vi "Drum SubviUpdated.vi"(8 "Image Dst Out":T2, 14 "error out":errorcluster) -> (7 "Red Drum":bool, 9 "Yellow Array":bool[](array[boolean]), 13 "Foot Pedal":bool, 16 "Blue array":bool[](array[boolean]), 17 "Red Array":bool[](array[boolean]), 20 "Green Array":bool[](array[boolean]), 23 "Blue Drum 2":bool, 24 "Yellow Drum":bool, 25 "Green Drum":bool, 27 "error out 2":errorcluster)   [LabVIEW 2009]
uses:
  <vilib>/vision/Image Controls.llb/IMAQ Image.ctl
  <vilib>/Analysis/3filter.llb/Filter Passband Type.ctl
  <vilib>/Analysis/3filter.llb/Butterworth Filter (DBL).vi
  <vilib>/Analysis/NI_AALBase.lvlib
  <vilib>/vision/NI_Vision_Development_Module.lvlib
panel:
  in  "Yellow Drum":T1={"Global Rectangle"=[40, 272, 657, 396], "Contours"=[{"ID"=enum."External", "Type"=3, "Coordinates"=[40, 272, 657, 396]}]} {"Contours"."Type" items=["No Selection", "Point", "Line", "Rectangle", "Oval", "Polygon", "Freehand Region", "Annulus", "Unused2", "Unused3", "Broken Line", "Freehand Line", "Rotated Rectangle"]}
  in  "Red Drum":T1={"Global Rectangle"=[40, 272, 657, 396], "Contours"=[{"ID"=enum."External", "Type"=3, "Coordinates"=[40, 272, 657, 396]}]} {"Contours"."Type" items=["No Selection", "Point", "Line", "Rectangle", "Oval", "Polygon", "Freehand Region", "Annulus", "Unused2", "Unused3", "Broken Line", "Freehand Line", "Rotated Rectangle"]}
  in  "Green Drum":T1={"Global Rectangle"=[40, 272, 657, 396], "Contours"=[{"ID"=enum."External", "Type"=3, "Coordinates"=[40, 272, 657, 396]}]} {"Contours"."Type" items=["No Selection", "Point", "Line", "Rectangle", "Oval", "Polygon", "Freehand Region", "Annulus", "Unused2", "Unused3", "Broken Line", "Freehand Line", "Rotated Rectangle"]}
  in  "Blue Drum":T1={"Global Rectangle"=[40, 272, 657, 396], "Contours"=[{"ID"=enum."External", "Type"=3, "Coordinates"=[40, 272, 657, 396]}]} {"Contours"."Type" items=["No Selection", "Point", "Line", "Rectangle", "Oval", "Polygon", "Freehand Region", "Annulus", "Unused2", "Unused3", "Broken Line", "Freehand Line", "Rotated Rectangle"]}
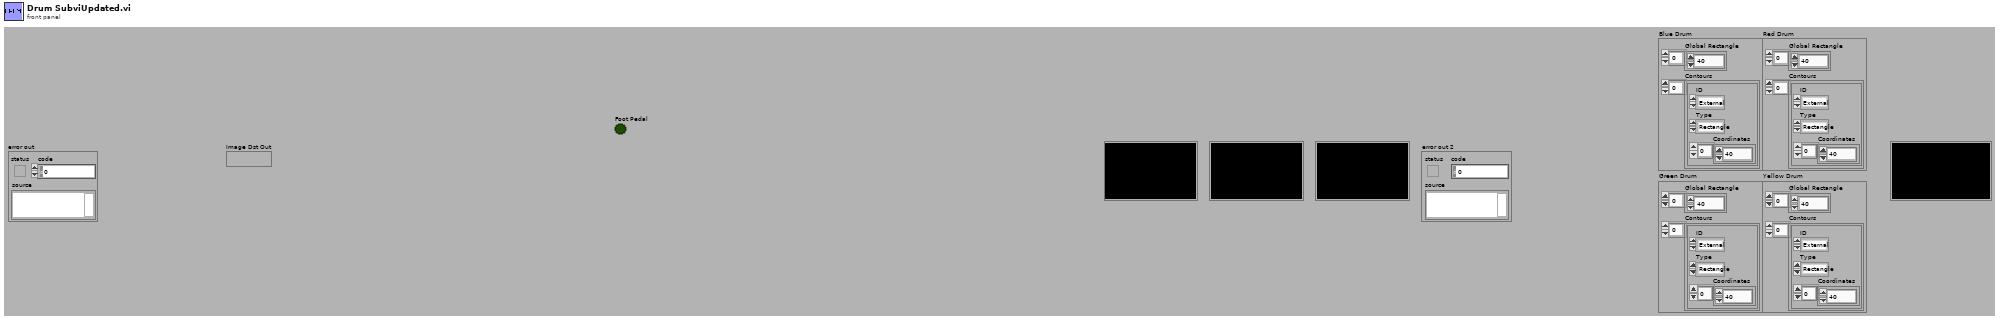
[diagram p1: front panel]
types:
  T1 = cluster{"Global Rectangle":i32[], "Contours":cluster{"ID":enum32{"External", "Internal"}, "Type":u32, "Coordinates":i32[]}[]}
  T2 = typedef "IMAQ Image.ctl" = refnum<image>
  T3 = typedef "NI_AALBase.lvlib/Filter Passband Type.ctl" = enum32{"Lowpass", "Highpass", "Bandpass", "Bandstop"}
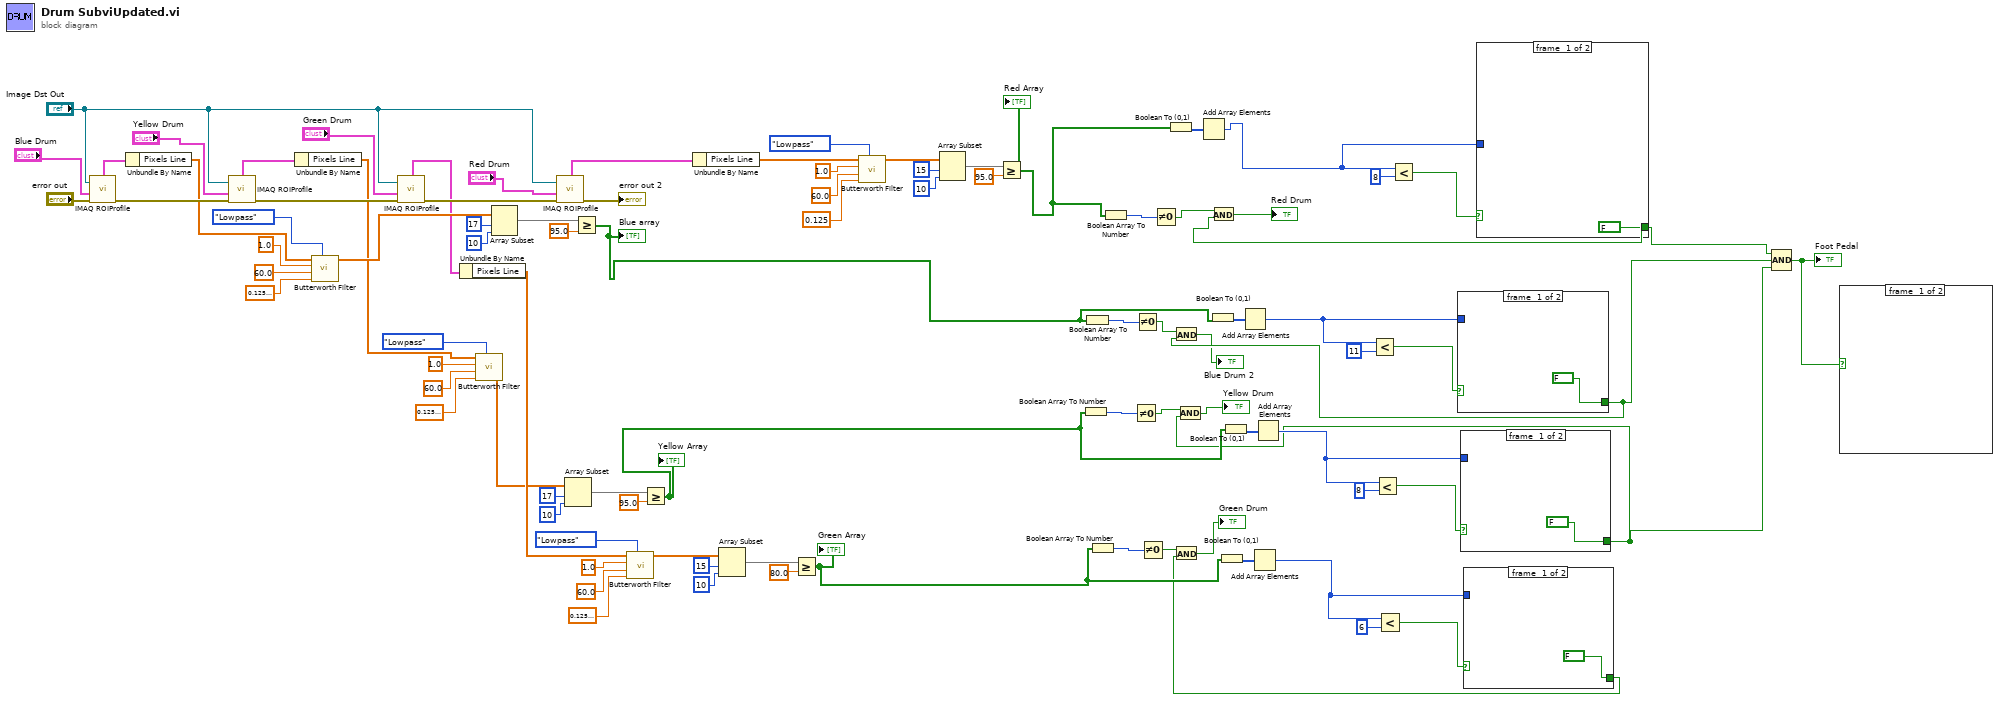
[diagram p0: block diagram]
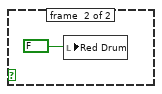
[diagram p2: hidden frame]
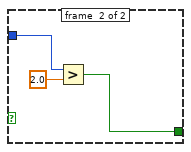
[diagram p3: hidden frame]
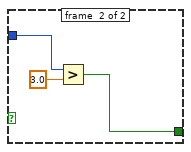
[diagram p4: hidden frame]
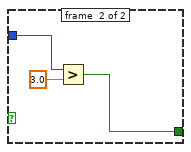
[diagram p5: hidden frame]
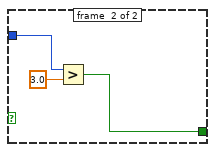
[diagram p6: hidden frame]
diagram:
  n1 = call "IMAQ ROIProfile"("error in (no error)"="error out", "ROI Descriptor"="Blue Drum", "Image"="Image Dst Out") -> ("error out"=w64:errorcluster, "ROI Graph"=w65:cluster{"x0":sgl, "dx":sgl, "Pixels Line":sgl[]})  [unwired: 4 out]
  n2 = Unbundle By Name(w65) -> ("Pixels Line"=w46:sgl[])
  n3 = call "IMAQ ROIProfile"("error in (no error)"=w64, "ROI Descriptor"="Yellow Drum", "Image"="Image Dst Out") -> ("error out"=w89:errorcluster, "ROI Graph"=w61:cluster{"x0":sgl, "dx":sgl, "Pixels Line":sgl[]})  [unwired: 4 out]
  n4 = Unbundle By Name(w61) -> ("Pixels Line"=w58:sgl[])
  n5 = call-poly <vilib>:"Butterworth Filter.vi"("filter type"=Filter_Passband_Type."Lowpass", "low cutoff freq: fl"=0.12500000000000006 ("low"), "high cutoff freq: fh"=60.0 ("high"), "sampling freq: fs"=1.0 ("sampling"), "X"=w46) -> ("Filtered X"=w77:dbl[])  [unwired: 3 in, 1 out]
  n6 = call "IMAQ ROIProfile"("error in (no error)"=w89, "ROI Descriptor"="Green Drum", "Image"="Image Dst Out") -> ("error out"=w88:errorcluster, "ROI Graph"=w67:cluster{"x0":sgl, "dx":sgl, "Pixels Line":sgl[]})  [unwired: 4 out]
  n7 = Unbundle By Name(w67) -> ("Pixels Line"=w70:sgl[])
  n8 = call-poly <vilib>:"Butterworth Filter.vi"("filter type"=Filter_Passband_Type."Lowpass", "low cutoff freq: fl"=0.12500000000000006 ("low  2"), "high cutoff freq: fh"=60.0 ("high 2"), "sampling freq: fs"=1.0 ("sampling 2"), "X"=w58) -> ("Filtered X"=w62:dbl[])  [unwired: 3 in, 1 out]
  n9 = Array Subset(array=w77, index=17, length=10) -> (w52:dbl[])
  n10 = call "IMAQ ROIProfile"("error in (no error)"=w88, "ROI Descriptor"="Red Drum", "Image"="Image Dst Out") -> ("error out"=→"error out 2":errorcluster, "ROI Graph"=w87:cluster{"x0":sgl, "dx":sgl, "Pixels Line":sgl[]})  [unwired: 4 out]
  n11 = Array Subset(array=w62, index=17, length=10) -> (w55:dbl[])
  n12 = Greater Or Equal?(x=w52, y=95.0) -> (x >= y?=w26:bool[])
  "Blue array" <- w26
  n13 = call-poly <vilib>:"Butterworth Filter.vi"("filter type"=Filter_Passband_Type."Lowpass", "low cutoff freq: fl"=0.12500000000000006 ("low  3"), "high cutoff freq: fh"=60.0 ("high 3"), "sampling freq: fs"=1.0 ("sampling 3"), "X"=w70) -> ("Filtered X"=w66:dbl[])  [unwired: 3 in, 1 out]
  n14 = Greater Or Equal?(x=w55, y=95.0) -> (x >= y?=w28:bool[])
  "Yellow Array" <- w28
  n15 = Unbundle By Name(w87) -> ("Pixels Line"=w84:sgl[])
  n16 = Array Subset(array=w66, index=15, length=10) -> (w73:dbl[])
  n17 = Greater Or Equal?(x=w73, y=80.0) -> (x >= y?=w30:bool[])
  "Green Array" <- w30
  n18 = call-poly <vilib>:"Butterworth Filter.vi"("filter type"=Filter_Passband_Type."Lowpass", "low cutoff freq: fl"=0.125 ("low  4"), "high cutoff freq: fh"=60.0 ("high 4"), "sampling freq: fs"=1.0 ("sampling 4"), "X"=w84) -> ("Filtered X"=w5:dbl[])  [unwired: 3 in, 1 out]
  n19 = Array Subset(array=w5, index=15, length=10) -> (w81:dbl[])
  n20 = Greater Or Equal?(x=w81, y=95.0) -> (x >= y?=w17:bool[])
  "Red Array" <- w17
  n21 = Boolean Array To Number(Boolean array=w28) -> (number=w41:u32)
  n22 = Boolean Array To Number(Boolean array=w26) -> (number=w42:u32)
  n23 = Boolean Array To Number(Boolean array=w30) -> (number=w40:u32)
  n24 = Boolean Array To Number(Boolean array=w17) -> (number=w18:u32)
  n25 = Not Equal To 0?(x=w41) -> (x != 0?=w15:bool)
  n26 = Not Equal To 0?(x=w42) -> (x != 0?=w13:bool)
  n27 = Not Equal To 0?(x=w40) -> (x != 0?=w14:bool)
  n28 = Not Equal To 0?(x=w18) -> (x != 0?=w16:bool)
  n29 = Boolean To (0,1)(Boolean=w17) -> (0, 1=w39:i16[])
  n30 = Add Array Elements(numeric array=w39) -> (sum=w36:i16)
  n31 = Boolean To (0,1)(Boolean=w26) -> (0, 1=w33:i16[])
  n32 = Boolean To (0,1)(Boolean=w30) -> (0, 1=w31:i16[])
  n33 = Boolean To (0,1)(Boolean=w28) -> (0, 1=w32:i16[])
  n34 = Add Array Elements(numeric array=w33) -> (sum=w25:i16)
  n35 = Add Array Elements(numeric array=w31) -> (sum=w29:i16)
  n36 = Add Array Elements(numeric array=w32) -> (sum=w27:i16)
  n37 = Less?(x=w25, y=i16 11) -> (x < y?=w35:bool)
  n38 = Less?(x=w27, y=i16 8) -> (x < y?=w24:bool)
  n39 = Less?(x=w29, y=i16 6) -> (x < y?=w21:bool)
  n40 = Less?(x=w36, y=i16 8) -> (x < y?=w37:bool)
  n41 = case shown="True" w35 {
    tunnel: w25 -> [_ w95]
    tunnel: [FALSE w94] -> w12
    frame #0 {
    }
    frame #1 {
      n42 = Greater?(x=w95, y=3.0) -> (0:w94:bool)
    }
  }
  n43 = And(x=w13, y=w12) -> (x .and. y?=→"Blue Drum 2":bool)
  n44 = case shown="True" w24 {
    tunnel: w27 -> [_ w99]
    tunnel: [FALSE w98] -> w10
    frame #0 {
    }
    frame #1 {
      n45 = Greater?(x=w99, y=3.0) -> (0:w98:bool)
    }
  }
  n46 = And(x=w15, y=w10) -> (x .and. y?=→"Yellow Drum":bool)
  n47 = case shown="True" w21 {
    tunnel: w29 -> [_ w103]
    tunnel: [FALSE w102] -> w7
    frame #0 {
    }
    frame #1 {
      n48 = Greater?(x=w103, y=2.0) -> (0:w102:bool)
    }
  }
  n49 = And(x=w14, y=w7) -> (x .and. y?=→"Green Drum":bool)
  n50 = case shown="True" w37 {
    tunnel: w36 -> [_ w106]
    tunnel: [FALSE w105] -> w20
    frame #0 {
    }
    frame #1 {
      n51 = Greater?(x=w106, y=3.0) -> (0:w105:bool)
    }
  }
  n52 = And(x=w16, y=w20) -> (x .and. y?=→"Red Drum":bool)
  n53 = Compound Arithmetic op=AND(w20, w12, w10) -> (w6:bool)
  "Foot Pedal" <- w6
  n54 = case shown="False" w6 {
    frame #0 {
    }
    frame #1 {
      n55 = local write "Red Drum"(FALSE) -> ()
    }
  }
